vi "PH_PPPA_PowerUnit.PC_StateTrigger.vi"(0 "i ref in":refnum<vi>, 2 "Trigger Status":T1 items=["no info", "off/false/out", "on/true/in", "Failure", "Alarm", "Status 1", "Status 2", "Status 3"], 3 "not linked?":bool, 5 "error in (no error)":errorcluster) -> (14 "i ref out":refnum<vi> caption="VI Refnum", 19 "error out":errorcluster)   [LabVIEW 2014, in "PH_PPPA_PowerUnit.lvlib"]
doc: "This VI writes the Trigger Tag Information to own attributes and sets the GUI object."
uses:
  PH_PPPA_PowerUnit.lvlib
  PH_Basics/PH_StatusHandler/PH_StatusHandler.Status.ctl
  PH_Basics/PH_Common/PH_Common.lvlib
  CS_Core/BaseSM/BaseSM.lvlib
  PH_Basics/PH_StatusHandler/PH_StatusHandler.lvlib
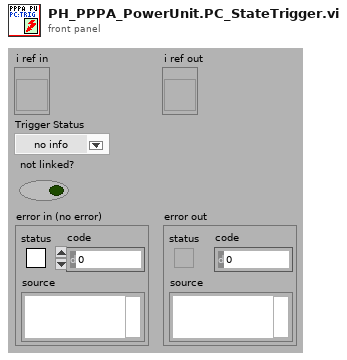
[diagram p1: front panel]
types:
  T1 = typedef "PH_StatusHandler.lvlib/PH_StatusHandler.Status.ctl" = i16
  T2 = typedef "PH_PPPA_PowerUnit.lvlib/PH_PPPA_PowerUnit.i attribute.ctl" = cluster{"GUI Refs":cluster{"Ignitron":refnum<vi>, "Rossrelais":refnum<vi>, "Set Voltage":refnum<vi>, "PSU":refnum<vi>, "EOC":refnum<vi>, "Trigger":refnum<vi>}, "Ignitron":T3, "PSU":T4, "Dump Ross Relais":T5, "Trigger":cluster{"State Device":T1, "linked?":bool}, "Timing Settings":cluster{"Prdc Fast?":bool, "Default Value Periodic Interval":i32, "Mercury on since":dbl, "Warm up Time Mercury [s]":dbl}, "Set Voltage [V]":dbl, "19er Ignitionbox":string}
  T3 = typedef "PH_PP_Common.lvlib/PH_PP_Common.Ignitron Attributes.ctl" = cluster{"State Device":T1, "linked?":bool}
  T4 = typedef "PH_PP_Common.lvlib/PH_PP_Common.PSU Attributes.ctl" = cluster{"lower limit [V]":dbl, "upper limit [V]":dbl, "Voltage set":bool, "State Device":T1, "linked?":bool}
  T5 = typedef "PH_PP_Common.lvlib/PH_PP_Common.Ross Relais Attributes.ctl" = cluster{"State Device":T1, "linked?":bool}
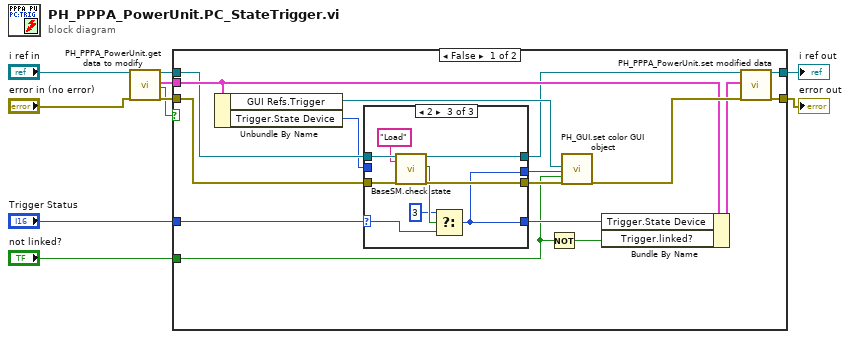
[diagram p0: block diagram]
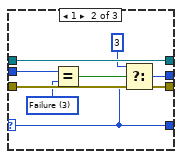
[diagram p3: hidden frame]
diagram:
  n1 = call "PH_PPPA_PowerUnit.get data to modify.vi"("i ref in"="i ref in", "error in (no error)"="error in (no error)") -> ("i ref out"=w6:refnum<vi>, "i attribute"=w4:T2, "timed out"=w3:bool, "error out"=w5:errorcluster)  [unwired: 14 in]
  n2 = case shown="False" w3 {
    tunnel: w6 -> [w18 w48]
    tunnel: [w12 w48] -> w9
    tunnel: w5 -> [w20 w47]
    tunnel: [w11 w47] -> w10
    tunnel: w4 -> [w24 _]
    tunnel: "Trigger Status" -> [w15 _]
    tunnel: "not linked?" -> [w14 _]
    frame False {
      n3 = Unbundle By Name(w24) -> ("GUI Refs.Trigger"=w23:refnum<vi>, "Trigger.State Device"=w16:T1)
      n4 = case shown="2" w15 {
        selector: w15 -> [w29 w31 w39]
        tunnel: [w29 w31 w40] -> w22
        tunnel: [w29 w32 w40] -> w21
        tunnel: w20 -> [w27 w36 w44]
        tunnel: [w27 w36 w43] -> w19
        tunnel: w18 -> [w28 w37 w46]
        tunnel: [w28 w37 w45] -> w17
        tunnel: w16 -> [_ w35 _]
        frame 0, Default {
        }
        frame 1 {
          w30 = T1 3 items=["no info", "off/false/out", "on/true/in", "Failure", "Alarm", "Status 1", "Status 2", "Status 3"] ("Trigger.State Device")
          n5 = Equal?(x=w35, y=w30) -> (x = y?=w34:bool)
          n6 = Select(t=3, s=w34, f=w31) -> (s? t:f=w32:i32)
        }
        frame 2 {
          n7 = call "BaseSM.check state.vi"("i ref in"=w46, "requestedState"="Load" ("requested state"), "error in (no error)"=w44) -> ("i ref out"=w45:refnum<vi>, "OK"=w41:bool, "error out"=w43:errorcluster)  [unwired: 11 in, 3 out]
          n8 = Select(t=3 ("f"), s=w41, f=w39) -> (s? t:f=w40:i32)
        }
      }
      n9 = Not(x=w14) -> (.not. x?=w13:bool)
      n10 = call "PH_GUI.set color GUI object.vi"("GUI object Ref"=w23, "State"=w21, "Blinking? (false)"=w14, "error in (no error)"=w19) -> ("error out"=w26:errorcluster)  [unwired: 15 in]
      n11 = Bundle By Name(cluster=w24, "Trigger.State Device"=w22, "Trigger.linked?"=w13) -> (w25:T2)
      n12 = call "PH_PPPA_PowerUnit.set modified data.vi"("i ref in"=w17, "i attribute"=w25, "error in (no error)"=w26) -> ("i ref out"=w12:refnum<vi>, "error out"=w11:errorcluster)  [unwired: 15 in]
    }
    frame True {
    }
  }
  "error out" <- w10
  "i ref out" <- w9
